vi "Load Module.vi"(8 "error in (no error)":errorcluster) -> (0 "error out":errorcluster)   [LabVIEW 2020, in "Event Manager.lvlib"]
doc: "Combines Start Module.vi and Synchronize Module Events.vi. Wrapping these allows to programmatically start any module (by use of call by reference) as the module-specific connector panes are hidden away.\n\n____\nHAMPEL SOFTWARE ENGINEERING v2.6.0 (2023-12-19 10:54)"
uses:
  Event Manager.lvlib
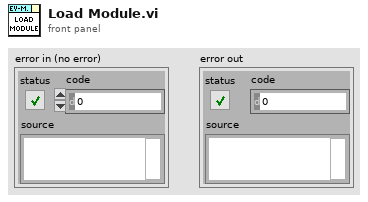
[diagram p1: front panel]
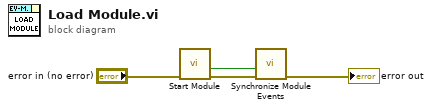
[diagram p0: block diagram]
diagram:
  n1 = call "Start Module.vi"("error in (no error)"="error in (no error)") -> ("error out"=w1:errorcluster, "Wait for Event Sync?"=w2:bool)  [unwired: 7 in, 2 out]
  n2 = call "Synchronize Module Events.vi"("error in (no error)"=w1, "Wait for Event Sync?"=w2) -> ("error out"=→"error out":errorcluster)  [unwired: 9 in]
